vi "Open.vi"(4 "ReceiveId":u32=1851 format="%08x", 5 "LogEnabled":bool, 6 "TransmittId":u32=1843 format="%08x", 7 "LogPath":path, 8 "error in":errorcluster {"code" format="%.0x"}, 10 "BaudRate":u32=125000, 11 "UdsHandleIn":T1) -> (0 "error out":errorcluster {"code" format="%.0x"}, 3 "UdsHandleOut":T1)   [LabVIEW 2011, in "Konvolucio MUDS150628.lvlib"]
uses:
  <instrlib>/Konvolucio MUDS150628/Konvolucio MUDS150628.lvlib
  <instrlib>/Konvolucio MUDS150628/Types/UdsHandleType.ctl
  <instrlib>/Konvolucio MCAN120803/Types/MCanHandleType.ctl
  C:/Program Files/National Instruments/LabVIEW 2011/instr.lib/Konvolucio MCAN120803/Private/Konvolucio.MCAN120803.dll
  Konvolucio MCAN120803/Private/Konvolucio.MCAN120803.dll
  <instrlib>/Konvolucio MUDS150628/Private/UdsLogEvent.vi
  <instrlib>/Konvolucio MCAN120803/Konvolucio MCAN120803.lvlib
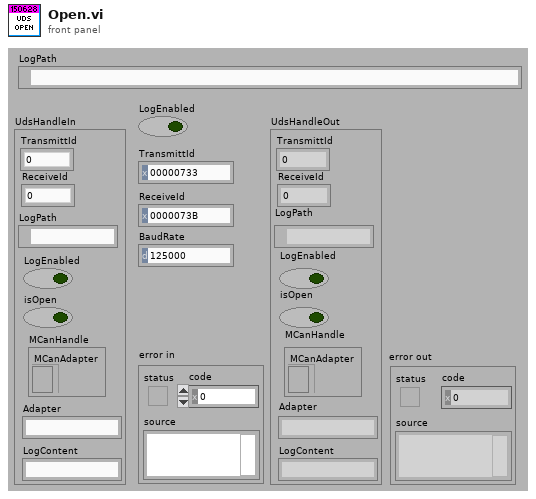
[diagram p1: front panel]
types:
  T1 = typedef "Konvolucio MUDS150628.lvlib/UdsHandleType.ctl" = cluster{"LogPath":path, "LogEnabled":bool, "isOpen":bool, "LogContent":string, "Adapter":string, "MCanHandle":T2, "TransmittId":u32, "ReceiveId":u32}
  T2 = typedef "Konvolucio MCAN120803.lvlib/MCanHandleType.ctl" = cluster{"MCanAdapter":refnum<k24>}
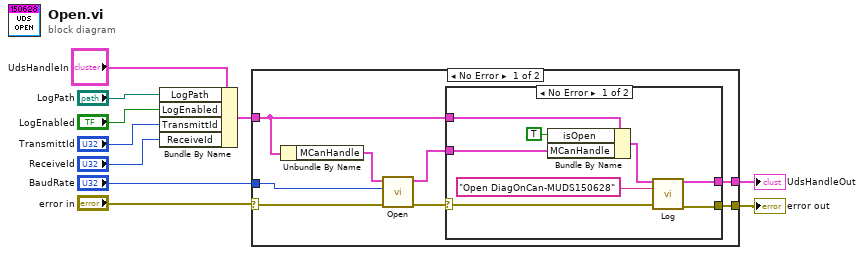
[diagram p0: block diagram]
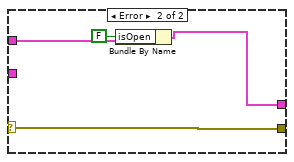
[diagram p2: hidden frame]
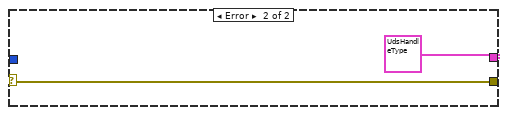
[diagram p3: hidden frame]
diagram:
  n1 = Bundle By Name(cluster="UdsHandleIn", "LogPath"="LogPath", "LogEnabled"="LogEnabled", "TransmittId"="TransmittId", "ReceiveId"="ReceiveId") -> (w3:T1)
  n2 = case shown="No Error" "error in" {
    selector: "error in" -> [w13 w32]
    tunnel: [w18 w32] -> w10
    tunnel: [w17 T1 {"LogPath"=path "", "LogEnabled"=FALSE, "isOpen"=FALSE, "LogContent"="", "Adapter"="", "MCanHandle"={"MCanAdapter"=refnum}, "TransmittId"=0, "ReceiveId"=0} ("HandlerIn")] -> w8
    tunnel: "BaudRate" -> [w14 _]
    tunnel: w3 -> [w11 _]
    frame No Error {
      n3 = Unbundle By Name(w11) -> ("MCanHandle"=w12:T2)
      n4 = call <instrlib>:"Open.vi"("error in"=w13, "Baudrate"=w14, "MCanHandleIn"=w12) -> ("error out"=w16:errorcluster, "MCanHandleOut"=w15:T2)  [unwired: 7 in]
      n5 = case shown="No Error" w16 {
        selector: w16 -> [w23 w30]
        tunnel: [w20 w30] -> w18
        tunnel: w11 -> [w25 w28]
        tunnel: [w21 w27] -> w17
        tunnel: w15 -> [w24 _]
        frame No Error {
          n6 = Bundle By Name(cluster=w25, "isOpen"=TRUE, "MCanHandle"=w24) -> (w22:T1)
          n7 = call-poly <instrlib>:"Log.vi"("UdsHandleIn"=w22, "EventMsg"="Open DiagOnCan-MUDS150628", "error in"=w23) -> ("UdsHandleOut"=w21:T1, "error out"=w20:errorcluster)  [unwired: 11 in]
        }
        frame Error {
          n8 = Bundle By Name(cluster=w28, "isOpen"=FALSE) -> (w27:T1)
        }
      }
    }
    frame Error {
    }
  }
  "error out" <- w10
  "UdsHandleOut" <- w8
